vi "de santimeters by encoder.vi"() -> ()   [LabVIEW 2017]
uses:
  <vilib>/myRIO/Express VI/Onboard IO/Encoder/Encoder Express VI.xnode
  <vilib>/myRIO/Instrument Drivers/Onboard IO/Encoder/vis/Read.vi
  <vilib>/myRIO/Instrument Drivers/Onboard IO/Encoder/Encoder.lvlib
  <vilib>/myRIO/Common/Instrument Driver Framework/myRIO v1.0/Encoder/typedefs/Encoder Signal Mode.ctl
  <vilib>/myRIO/Common/Instrument Driver Framework/myRIO v1.0/Encoder/typedefs/Encoder Channels Enum.ctl
  <vilib>/myRIO/Common/Instrument Driver Framework/Utilities/typedefs/Generic FPGA Reference.ctl
  <vilib>/myRIO/Common/Instrument Driver Framework/Utilities/typedefs/myRIO v1.0 Reference.ctl
  <vilib>/myRIO/Common/Instrument Driver Framework/Utilities/typedefs/Hardware Version Enum.ctl
  <vilib>/myRIO/Common/Instrument Driver Framework/Utilities/typedefs/myRIO Generic Hardware Reference.ctl
  <vilib>/myRIO/Instrument Drivers/Onboard IO/Encoder/typedefs/Encoder Reference.ctl
  <vilib>/myRIO/Instrument Drivers/Onboard IO/Encoder/vis/myRIO Encoder Open.xnode
  <vilib>/myRIO/Common/Instrument Driver Framework/Utilities/vis/Is FPGA Ref Available.vi
  <vilib>/myRIO/Common/Instrument Driver Framework/myRIO v1.0/Encoder/vis/myRIO v1.1 Open Encoder.vi
  <vilib>/myRIO/Common/Instrument Driver Framework/myRIO v1.0/Encoder/vis/myRIO v1.0 Configure Encoder.vi
  <vilib>/myRIO/Common/Instrument Driver Framework/myRIO v1.0/Encoder/typedefs/Encoder Configuration v1.0.ctl
  <vilib>/userdefined/High Color/nirio_resource_hc.ctl
  <vilib>/myRIO/Instrument Drivers/Utilities/Utilities.lvlib
panel:
  out "curret value":i32
  in  "Stop Button":bool
  in  "range":dbl format="%#_13g"
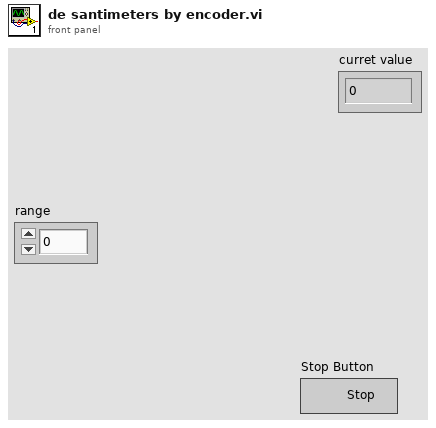
[diagram p1: front panel]
types:
  T1 = typedef "Encoder.lvlib/Encoder Reference.ctl" = cluster{"myRIO Reference":T2, "Encoder Channels Enum":T6}
  T2 = typedef "myRIO Generic Hardware Reference.ctl" = cluster{"myRIO Model":T3, "myRIO Hardware Reference":T4}
  T3 = typedef "Hardware Version Enum.ctl" = enum16{"Unknown", "myRIO-1900", "myRIO-1950", "roboRIO", "NI ELVIS RIO CM"}
  T4 = typedef "myRIO v1.0 Reference.ctl" = cluster{"Generic FPGA Reference":T5, "Allow multiple opens":bool}
  T5 = typedef "Generic FPGA Reference.ctl" = refnum<k20>
  T6 = typedef "Encoder Channels Enum.ctl" = enum16{"Not Connected", "C/ENC0", "C/ENC1", "A/ENC", "B/ENC", "DIO/ENC0", "DIO/ENC1", "DIO/ENC2", "DIO/ENC3", "DIO/ENC4"}
  T7 = typedef "Encoder Signal Mode.ctl" = enum16{"Quadrature phase signal", "Step and direction signal"}
  T8 = typedef "nirio_resource_hc.ctl" = tag
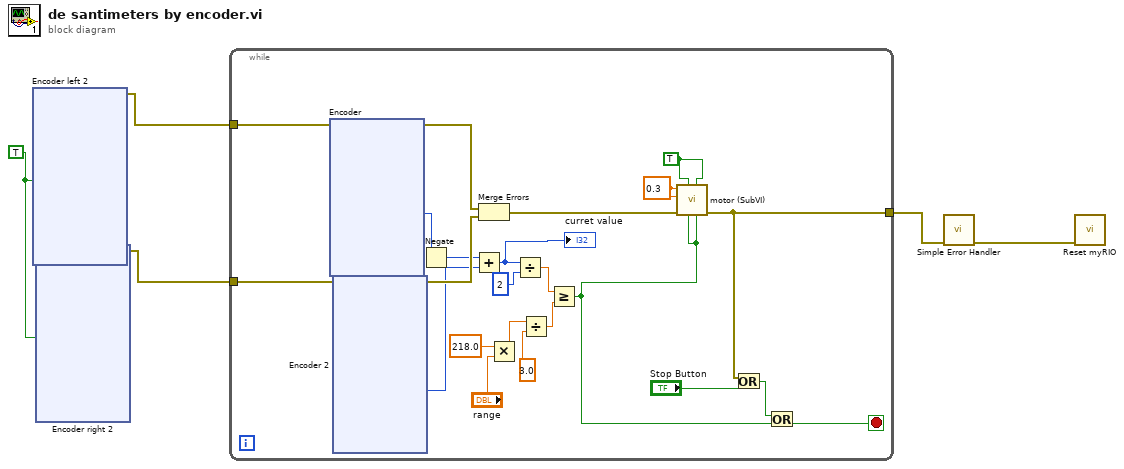
[diagram p0: block diagram]
diagram:
  w3 = TRUE ("Reset Counter")
  n1 = xnode "Encoder left 2"("Reset Counter"=w3) -> ("error out"=w2:errorcluster)  [unwired: 1 in, 3 out]
  n2 = xnode "Encoder right 2"("Reset Counter"=w3) -> ("error out"=w1:errorcluster)  [unwired: 1 in, 3 out]
  n3 = while {
    tunnel: [w14] -> w5
    tunnel: w2 -> [w13]
    tunnel: w1 -> [w12]
    stop <- w20 stop-if-true
    w16 = TRUE
    w17 = 0.3 ("PWM0")
    n4 = xnode "Encoder"("error in (no error)"=w13) -> ("Counter Value"=w25:i32, "error out"=w27:errorcluster)  [unwired: 1 in, 2 out]
    n5 = xnode "Encoder 2"("error in (no error)"=w12) -> ("Counter Value"=w24:i32, "error out"=w26:errorcluster)  [unwired: 1 in, 2 out]
    n6 = Negate(x=w25) -> (-x=w11:i32)
    n7 = Add(x=w11, y=w24) -> (x+y=w10:i32)
    "curret value" <- w10
    n8 = Merge Errors(w27, w26) -> (w28:errorcluster)
    n9 = Multiply(x=218.0, y="range") -> (x*y=w7:dbl)
    n10 = Divide(x=w10, y=2) -> (x/y=w22:dbl)
    n11 = Divide(x=w7, y=3.0) -> (x/y=w8:dbl)
    n12 = Greater Or Equal?(x=w22, y=w8) -> (x >= y?=w15:bool)
    n13 = call "motor (SubVI).vi"("M1 (Pin 26)"=w15, "M1 (Pin 25)"=w16, "M0 (Pin 23)"=w15, "M0 (Pin 21)"=w16, "error in (no error)"=w28, "PWM1"=w17, "PWM0"=w17) -> ("error out"=w14:errorcluster)  [unwired: 4 in]
    n14 = Or(x=w14, y="Stop Button") -> (x .or. y?=w19:bool)
    n15 = Or(x=w19, y=w15) -> (x .or. y?=w20:bool)
  }
  n16 = call <vilib>:"Simple Error Handler.vi"("error in (no error)"=w5) -> ("error out"=w4:errorcluster)  [unwired: 4 in, 4 out]
  n17 = call <vilib>:"Reset myRIO.vi"("error in (no error)"=w4) -> ()  [unwired: 10 in, 1 out]
